vi "Release Control Cluster.vi"(11 "output cluster":T1={"I-O.lvclass"=refnum, "Motion.lvclass"=refnum, "Dispenser.lvclass"=refnum}) -> ()   [LabVIEW 2016, in "Controller.lvclass"]
uses:
  Controller.lvclass
  Controllers.ctl
  I-O/I-O.lvclass
  Motion/A3200/A3200.lvclass
  Dispenser/Dispenser.lvclass
  Motion/Motion.lvclass
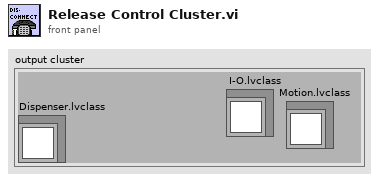
[diagram p1: front panel]
types:
  T1 = typedef "Controller.lvclass/Controllers.ctl" = cluster{"I-O.lvclass":refnum<class "I-O.lvclass">, "Motion.lvclass":refnum<class "Motion.lvclass">, "Dispenser.lvclass":refnum<class "Dispenser.lvclass">}
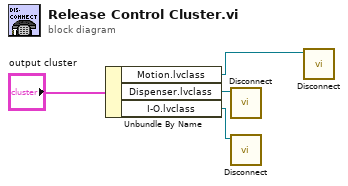
[diagram p0: block diagram]
diagram:
  n1 = Unbundle By Name("output cluster") -> ("Motion.lvclass"=w3:refnum<class "Motion.lvclass">, "Dispenser.lvclass"=w1:refnum<class "Dispenser.lvclass">, "I-O.lvclass"=w2:refnum<class "I-O.lvclass">)
  n2 = call-dynamic "Disconnect.vi"("Controller in"=w1) -> ()  [unwired: 9 in, 1 out]
  n3 = call-dynamic "Disconnect.vi"("I-O in"=w2) -> ()  [unwired: 9 in, 1 out]
  n4 = call-dynamic "Disconnect.vi"("Controller in"=w3) -> ()  [unwired: 9 in, 1 out]
